vi "Write 3D Comet Property Array.vi"(8 "error in (no error)":errorcluster, 10 "3D Comet Property Array":T1, 11 "3D Comet.lvclass in":refnum<class "3D Comet.lvclass">) -> (0 "error out":errorcluster, 3 "3D Comet.lvclass out":refnum<class "3D Comet.lvclass">)   [LabVIEW 2017, in "3D Comet.lvclass"]
uses:
  <vilib>/Math Plots/3D Math Plots/3D Comet/3D Comet/3D Comet.lvclass
  <vilib>/Math Plots/3D Math Plots/3D Comet/3D Comet/Typedef/3D Comet Property Array.ctl
  <vilib>/Math Plots/3D Math Plots/3D Comet/3D Comet/Typedef/3D Comet Property.ctl
  <vilib>/Math Plots/3D Math Plots/3D Plot/3D Plot/Typedef/Sprite Type.ctl
  <vilib>/Math Plots/3D Math Plots/3D Plot/3D Plot/Typedef/Line Type.ctl
  <vilib>/Math Plots/3D Math Plots/3D Comet/3D Comet/3D Comet.lvclass/3D Comet.ctl
  <vilib>/Math Plots/3D Math Plots/3D Plot/3D Plot/3D Plot.lvclass
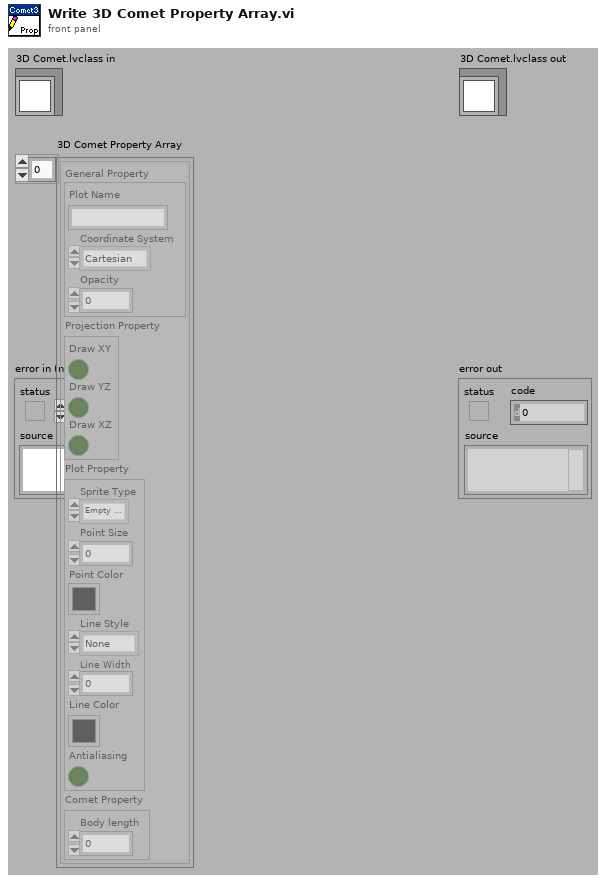
[diagram p1: front panel]
types:
  T1 = typedef "3D Comet.lvclass/3D Comet Property Array.ctl" = T2[]
  T2 = typedef "3D Comet.lvclass/3D Comet Property.ctl" = cluster{"General Property":cluster{"Plot Name":string, "Coordinate System":enum16{"Cartesian", "Cylindrical", "Spherical"}, "Opacity":sgl}, "Projection Property":cluster{"Draw XY":bool, "Draw YZ":bool, "Draw XZ":bool}, "Plot Property":cluster{"Sprite Type":T3, "Point Size":sgl, "Point Color":u32, "Line Style":T4, "Line Width":sgl, "Line Color":u32, "Antialiasing":bool}, "Comet Property":cluster{"Body length":sgl}}
  T3 = typedef "3D Plot.lvclass/Sprite Type.ctl" = enum16{"None", "Empty Square", "Solid Square", "Empty Diamond", "Solid Diamond", "Empty Circle", "Solid Circle", "Asterisk", "Bold X", "Wireframe Sphere", "Solid Sphere", "Wireframe Cube", "Solid Cube"}
  T4 = typedef "3D Plot.lvclass/Line Type.ctl" = enum16{"None", "Solid", "Dash", "Dot", "Dash Dot"}
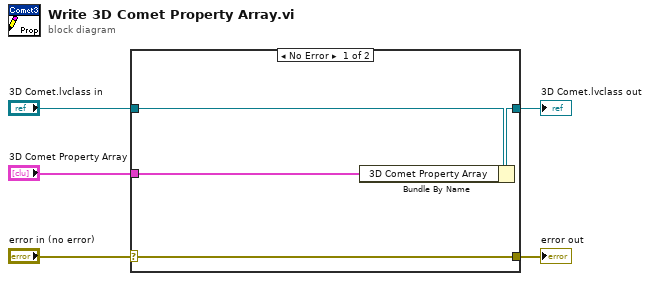
[diagram p0: block diagram]
diagram:
  n1 = case shown="No Error" "error in (no error)" {
    selector: "error in (no error)" -> [w9 w10]
    tunnel: [w9 w10] -> w4
    tunnel: [w7 w11] -> w2
    tunnel: "3D Comet.lvclass in" -> [w8 w11]
    tunnel: "3D Comet Property Array" -> [w6 _]
    frame No Error {
      n2 = Bundle By Name(cluster=w8, "3D Comet Property Array"=w6) -> (w7:refnum<class "3D Comet.lvclass">)
    }
    frame Error {
    }
  }
  "error out" <- w4
  "3D Comet.lvclass out" <- w2
